vi "Run VI Dynamically2.vi"(8 "error in (no error)":errorcluster, 10 "Show FP?":bool, 11 "Vi Path":path) -> (0 "error out":errorcluster, 3 "vi reference":refnum<vi>)   [LabVIEW 2025]
doc: "Runs VI specified in path."
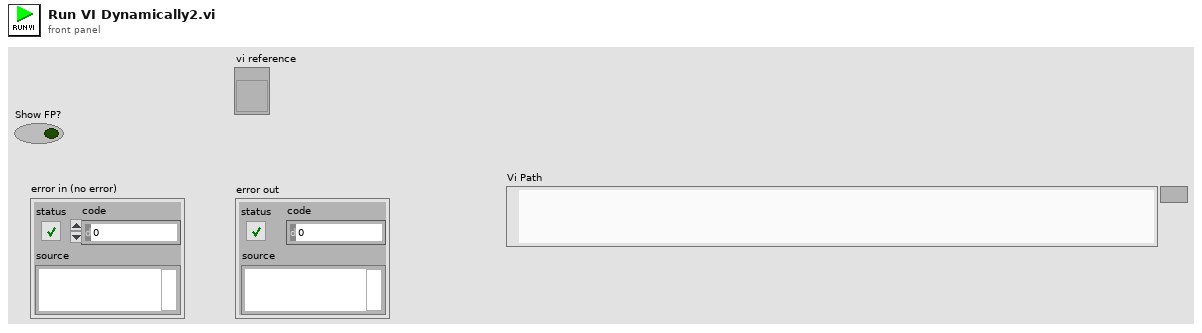
[diagram p1: front panel]
types:
  T1 = enum32{"Bad", "Idle", "Run top level", "Running"}
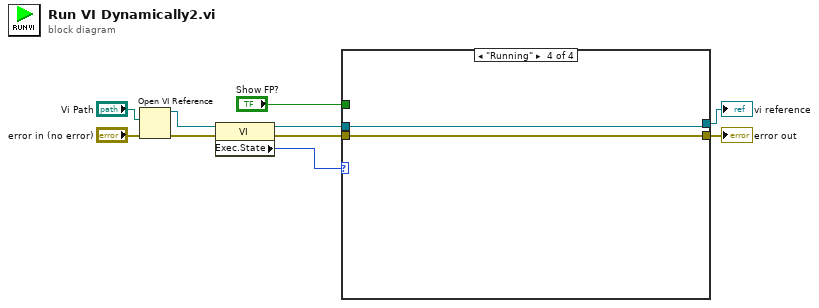
[diagram p0: block diagram]
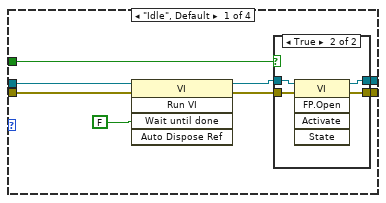
[diagram p2: hidden frame]
diagram:
  n1 = Open VI Reference(vi path="Vi Path", error in (no error)="error in (no error)") -> (vi reference=w6:refnum<vi>, error out=w4:errorcluster)  [unwired: 4 in]
  n2 = property class="VI"(reference=w6, error in=w4) -> (reference out=w5:refnum<vi>, error out=w3:errorcluster, "Exec.State"=w2:T1)
  n3 = case shown="\"Running\"" w2 {
    tunnel: [w17 w25 w27 w29] -> w10
    tunnel: [w15 w26 w28 w30] -> w7
    tunnel: w5 -> [w13 w26 w28 w30]
    tunnel: w3 -> [w12 w25 w27 w29]
    tunnel: "Show FP?" -> [w11 _ _ _]
    frame "Idle", Default {
      n4 = invoke on="Invoke Node" class="VI" method="Run VI"(reference=w13, error in=w12, "Wait until done"=FALSE ("Wait Until Done")) -> (reference out=w18:refnum<vi>, error out=w16:errorcluster)  [unwired: 2 in, 3 out]
      n5 = case shown="True" w11 {
        tunnel: w16 -> [w20 w24]
        tunnel: [w20 w23] -> w17
        tunnel: w18 -> [w19 w22]
        tunnel: [w19 w21] -> w15
        frame False {
        }
        frame True {
          n6 = invoke class="VI" method="FP.Open"(reference=w22, error in=w24) -> (reference out=w21:refnum<vi>, error out=w23:errorcluster)  [unwired: 3 in, 3 out]
        }
      }
    }
    frame "Bad" {
    }
    frame "Run top level" {
    }
    frame "Running" {
    }
  }
  "error out" <- w10
  "vi reference" <- w7
